vi "penning.vi"() -> ()   [LabVIEW 2014, in "Panels.lvlib"]
uses:
  Panels.lvlib
  CSlibraries-extern/DimLVEvent/DimIndicators/DimIndicators.lvlib
  CSlibraries/UtilityLib/UtilityLib.lvlib
  CSCore/CSSystem/CoreLib/CoreLib.lvlib
  CSlibraries/UtilityLib/UtilityLib.valueStatus.ctl
  Instance           1 15Saved   penning .vi
  CSCore/CSSystem/CoreLib/CoreLib.double 2 byte array.vi
  CSCore/CSSystem/CoreLib/CoreLib.string 2 byte array.vi
  CSlibraries-extern/DimLVEvent/LVDimInterface/LVDimInterface.lvlib
  CSCore/CSSystem/CoreLib/CoreLib.short 2 byte array.vi
  CSlibraries-extern/DimLVEvent/DimIndicators/DimIndicators.numericType.ctl
  CSCore/BaseProcess/BaseProcess.descriptor string definition.ctl
  CSCore/BaseProcess/BaseProcess.lvlib
  CSCore/CSSystem/CoreDefs/CoreDefs.rawDataType.ctl
  CSCore/CSSystem/CoreDefs/CoreDefs.call_type.ctl
  CSlibraries-extern/DimLVEvent/DimIndicators/DimIndicators.numericArrayType.ctl
  CSlibraries-extern/DimLVEvent/DimIndicators/DimIndicators.anyType.ctl
panel:
  in  "ListOfBases_Data":T1={"data"="NOLINK", "no link"=TRUE, "quality"=-1, "timeStamp"=0.0}
  in  "SetFileLocation_Data":T1={"data"="NOLINK", "no link"=TRUE, "quality"=-1, "timeStamp"=0.0}
  in  "call cluster in":T2={"Object"="", "Selector"="", "CallType"=enum."synchronous", "Async Object"="", "Async Selector"="", "Data Descriptor"="", "Data"=[], "Error #"=0, "Expire"=0}
  in  "CorrRingPara":dbl
  in  "CorrTubePara":dbl
  out "i ref out 2":refnum<vi>
  in  "i ref in":refnum<vi>
  in  "PT Viewer":bool
  in  "HypEndcapBEj":bool
  in  "HypRing":bool
  in  "HypCorrTubeBEj":bool
  in  "HypCorrTubeBInj":bool
  in  "HypCorrTubeAEj":bool
  in  "HypCorrTubeAInj":bool
  in  "HypEndcapAEj":bool
  in  "HypEndcapATrap":bool
  in  "HypEndcapAInj":bool
  in  "HypEndcapBInj":bool
  in  "HypEndcapBTrap":bool
  in  "HypEndcapAInj_SetValueInfoData":T5={"data"=[-121.4, 120.2, 1.0], "no link"=FALSE, "quality"=0, "timeStamp"=3268846606.097}
  in  "HypEndcapAInj_SetData":T5={"data"=[0.0, 0.0, 0.0, 0.0], "no link"=FALSE, "quality"=1, "timeStamp"=3268846604.644}
  in  "HypRing_MonData":T6={"data"=inf, "no link"=FALSE, "quality"=1, "timeStamp"=3268846606.097}
  in  "HypCorrRingB_MonData":T6={"data"=inf, "no link"=FALSE, "quality"=1, "timeStamp"=3268846606.097}
  in  "HypEndcapBTrap_MonData":T6={"data"=inf, "no link"=FALSE, "quality"=1, "timeStamp"=3268846606.082}
  in  "HypCorrTubeBTrap_MonData":T6={"data"=inf, "no link"=FALSE, "quality"=1, "timeStamp"=3268846606.082}
  in  "HypCorrRingA_MonData":T6={"data"=inf, "no link"=FALSE, "quality"=1, "timeStamp"=3268846606.097}
  in  "HypCorrTubeATrap_MonData":T6={"data"=inf, "no link"=FALSE, "quality"=1, "timeStamp"=3268846606.082}
  in  "HypEndcapATrap_MonData":T6={"data"=inf, "no link"=FALSE, "quality"=1, "timeStamp"=3268846606.097}
  in  "HypEndcapATrap_SetValueInfoData":T5={"data"=[-121.3, 120.5, 1.0], "no link"=FALSE, "quality"=0, "timeStamp"=3268846606.082}
  in  "HypEndcapAEj_SetValueInfoData":T5={"data"=[-120.0, 120.0, 1.0], "no link"=FALSE, "quality"=0, "timeStamp"=3268846606.097}
  in  "HypEndcapATrap_SetData":T5={"data"=[0.0, 0.0, 0.0, 0.0], "no link"=FALSE, "quality"=1, "timeStamp"=3268846604.629}
  in  "HypEndcapAEj_SetData":T5={"data"=[0.0, 0.0, 0.0, 0.0], "no link"=FALSE, "quality"=1, "timeStamp"=3268846604.644}
  in  "HypCorrTubeAEj_SetData":T5={"data"=[0.0, 0.0, 0.0, 0.0], "no link"=FALSE, "quality"=1, "timeStamp"=3268846604.644}
  in  "PenningBase_SetValueInfoData":T5={"data"=[0.0, 10.0, -1.0], "no link"=FALSE, "quality"=0, "timeStamp"=3268846606.097}
  in  "HypCorrTubeBInj_SetValueInfoData":T5={"data"=[-119.8, 119.3, 1.0], "no link"=FALSE, "quality"=0, "timeStamp"=3268846606.082}
  in  "PenningBase_SetData":T5={"data"=[0.0, 0.0, 0.0, 0.0], "no link"=FALSE, "quality"=1, "timeStamp"=3268846604.91}
  out "HypCorrTubeBTrap_Mon":dbl=inf caption="HypCorrTubeB_Mon" format="%.4f"
  out "HypCorrRingA_Mon":dbl=inf format="%.4f"
  out "HypRing_Mon":dbl=inf format="%.4f"
  in  "HypCorrTubeBEj_SetValueInfoData":T5={"data"=[-120.0, 120.0, 1.0], "no link"=FALSE, "quality"=0, "timeStamp"=3268846606.097}
  in  "HypCorrTubeBInj_SetData":T5={"data"=[0.0, 0.0, 0.0, 0.0], "no link"=FALSE, "quality"=1, "timeStamp"=3268846604.66}
  in  "HypEndcapBEj_SetValueInfoData":T5={"data"=[-120.0, 120.0, 1.0], "no link"=FALSE, "quality"=0, "timeStamp"=3268846606.082}
  in  "HypCorrTubeBEj_SetData":T5={"data"=[0.0, 0.0, 0.0, 0.0], "no link"=FALSE, "quality"=1, "timeStamp"=3268846604.676}
  out "HypCorrTubeATrap_Mon":dbl=inf format="%.4f"
  out "i ref out":refnum<vi>
  in  "Last Loaded File_Data":T1={"data"="NOLINK", "no link"=TRUE, "quality"=-1, "timeStamp"=0.0}
  out "FileUpToDate":bool=TRUE caption="Parameter Changed"
  in  "Close All Panels":bool
  in  "HypCorrTubeAInj_SetValueInfoData":T5={"data"=[-120.6, 119.6, 1.0], "no link"=FALSE, "quality"=0, "timeStamp"=3268846606.082}
  in  "HypRing_SetValueInfoData":T5={"data"=[-121.0, 119.7, 1.0], "no link"=FALSE, "quality"=0, "timeStamp"=3268846606.082}
  in  "CorrRingPara_SetValueInfoData":T5={"data"=[0.0, 1.0, -1.0], "no link"=FALSE, "quality"=0, "timeStamp"=3268846606.097}
  in  "CorrTubePara_SetValueInfoData":T5={"data"=[0.0, 1.0, -1.0], "no link"=FALSE, "quality"=0, "timeStamp"=3268846606.097}
  in  "HypEndcapBInj_SetValueInfoData":T5={"data"=[-120.5, 119.4, 1.0], "no link"=FALSE, "quality"=0, "timeStamp"=3268846606.097}
  in  "HypEndcapBTrap_SetValueInfoData":T5={"data"=[-120.6, 119.9, 1.0], "no link"=FALSE, "quality"=0, "timeStamp"=3268846606.082}
  in  "HypCorrTubeAEj_SetValueInfoData":T5={"data"=[-120.0, 120.0, 1.0], "no link"=FALSE, "quality"=0, "timeStamp"=3268846606.082}
  in  "HypEndcapBTrap_SetData":T5={"data"=[0.0, 0.0, 0.0, 0.0], "no link"=FALSE, "quality"=1, "timeStamp"=3268846604.644}
  in  "HypEndcapBInj_SetData":T5={"data"=[0.0, 0.0, 0.0, 0.0], "no link"=FALSE, "quality"=1, "timeStamp"=3268846604.66}
  in  "CorrTubePara_SetData":T5={"data"=[0.0, 0.0, 0.0, 0.0], "no link"=FALSE, "quality"=1, "timeStamp"=3268846604.894}
  in  "CorrRingPara_SetData":T5={"data"=[0.0, 0.0, 0.0, 0.0], "no link"=FALSE, "quality"=1, "timeStamp"=3268846604.894}
  in  "HypRing_SetData":T5={"data"=[0.0, 0.0, 0.0, 0.0], "no link"=FALSE, "quality"=1, "timeStamp"=3268846604.644}
  in  "HypCorrTubeAInj_SetData":T5={"data"=[0.0, 0.0, 0.0, 0.0], "no link"=FALSE, "quality"=1, "timeStamp"=3268846604.644}
  in  "HypEndcapBEj_SetData":T5={"data"=[0.0, 0.0, 0.0, 0.0], "no link"=FALSE, "quality"=1, "timeStamp"=3268846604.644}
  in  "call cluster in":T2={"Object"="", "Selector"="", "CallType"=enum."synchronous", "Async Object"="", "Async Selector"="", "Data Descriptor"="", "Data"=[], "Error #"=0, "Expire"=0}
  in  "PenningBase":dbl
  out "Last Loaded File":string
  in  "SetFileLocation":path=path "\\\\intranet\\Files/projects/lebit/Data Exchange/data/PenningControl"
  out "HypCorrRingB_Mon":dbl=inf format="%.4f"
  out "HypEndcapATrap_Mon":dbl=inf format="%.4f"
  out "HypEndcapBTrap_Mon":dbl=inf format="%.4f"
  # "Parameter changed, data file is no longer up-to-date."
  # "HypCorrRingA"
  # "HypCorrRingB"
  # "HypEndcapA"
  # "HypEndcapB"
  # "HypCorrTubeA"
  # "HypCorrTubeB"
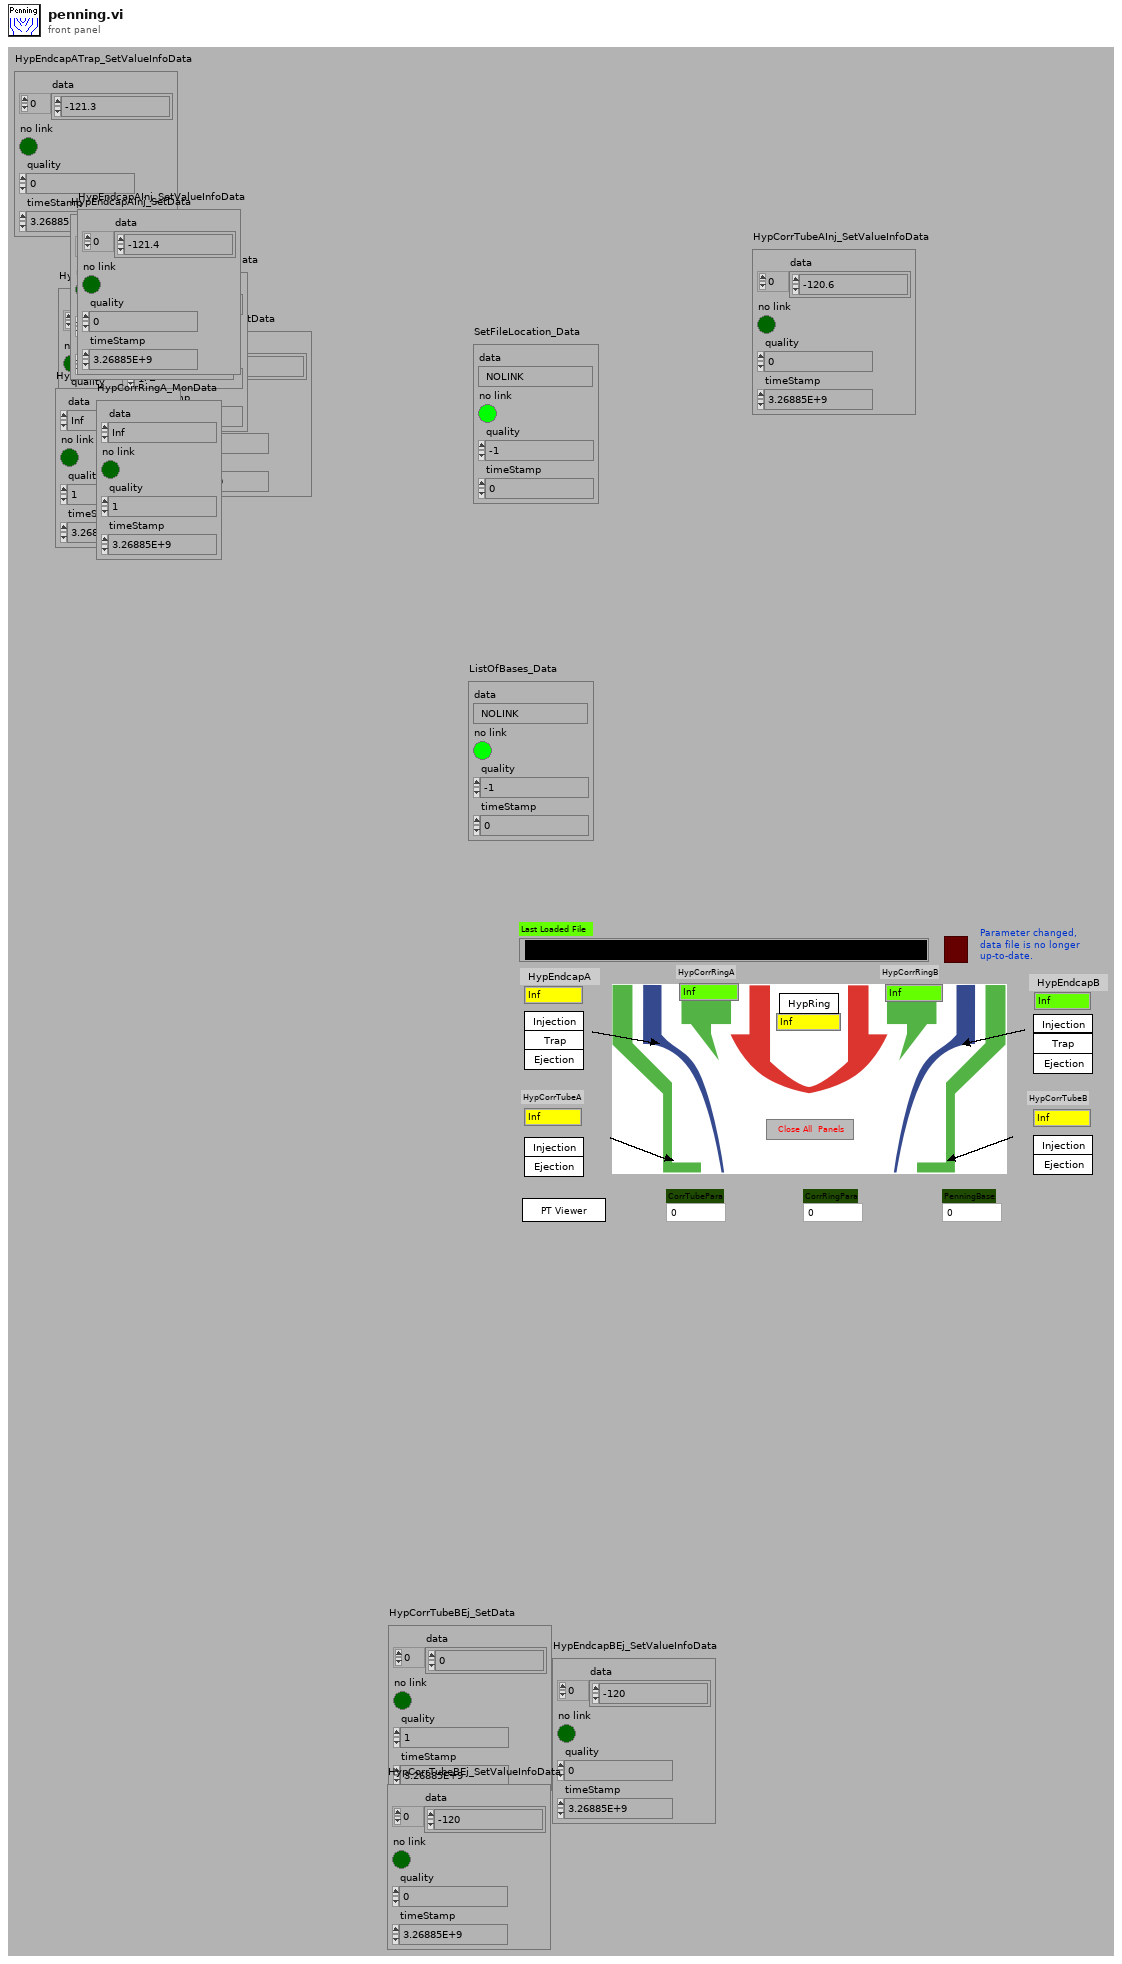
[diagram p1: front panel]
types:
  T1 = typedef "DimIndicators.lvlib/DimIndicators.anyType.ctl" = cluster{"data":string, "no link":bool, "quality":i32, "timeStamp":dbl}
  T2 = typedef "CoreDefs.call_type.ctl" = cluster{"Object":string, "Selector":string, "CallType":enum16{"simple", "synchronous", "asynchronous"}, "Async Object":string, "Async Selector":string, "Data Descriptor":T3, "Data":T4, "Error #":i32, "Expire":u32}
  T3 = typedef "BaseProcess.lvlib/BaseProcess.descriptor string definition.ctl" = string
  T4 = typedef "CoreDefs.rawDataType.ctl" = i8[]
  T5 = typedef "DimIndicators.lvlib/DimIndicators.numericArrayType.ctl" = cluster{"data":dbl[], "no link":bool, "quality":i32, "timeStamp":dbl}
  T6 = typedef "DimIndicators.lvlib/DimIndicators.numericType.ctl" = cluster{"data":dbl, "no link":bool, "quality":i32, "timeStamp":dbl}
  T7 = typedef "UtilityLib.lvlib/UtilityLib.valueStatus.ctl" = enum16{"no info available", "stand by/off", "on", "warning", "alarm/malfunction", "not implemented", "user action required", "important information", "system default", "control default", "indicator default", "button default"}
  T8 = cluster{"data":string, "no link":bool, "quality":i32, "timeStamp":dbl}
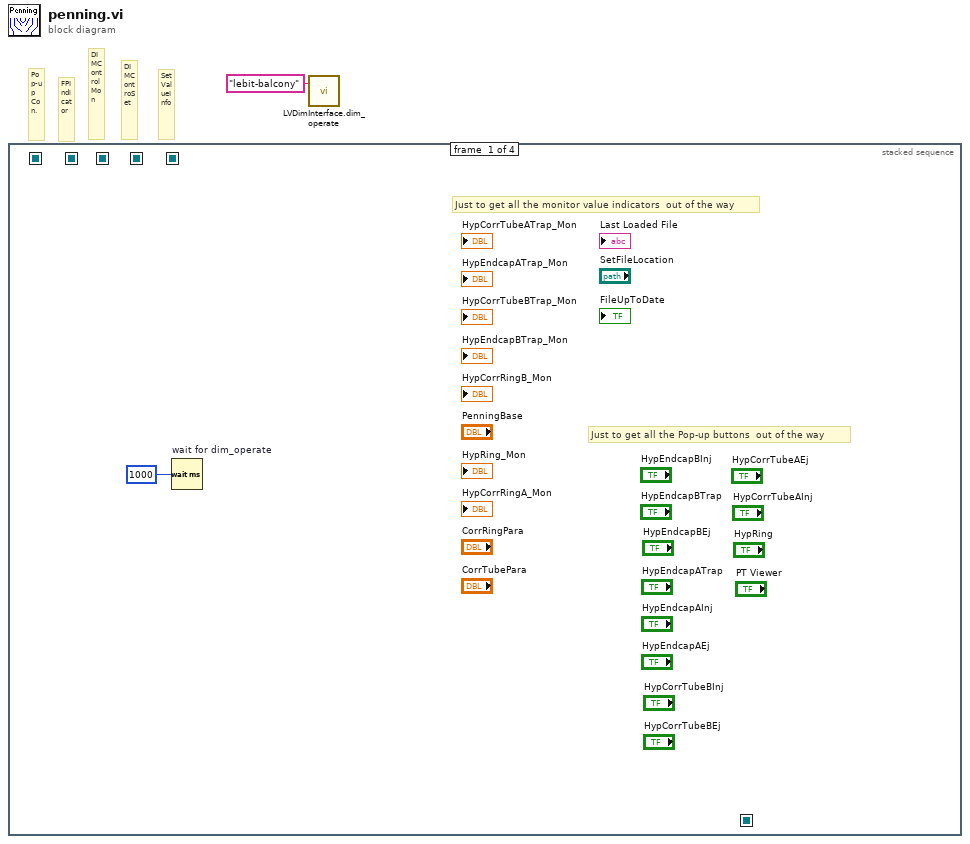
[diagram p0: block diagram]
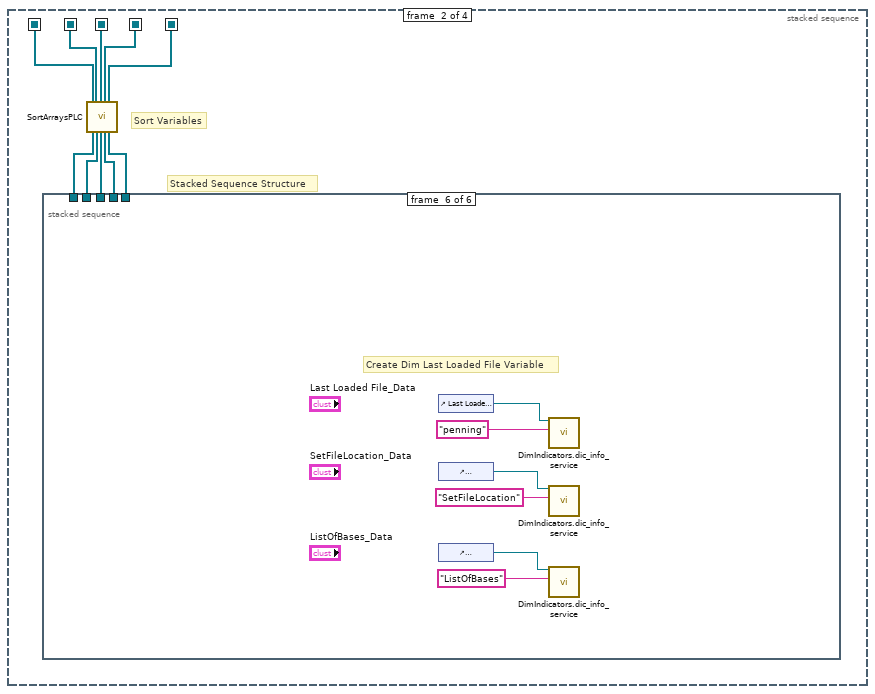
[diagram p2: hidden frame]
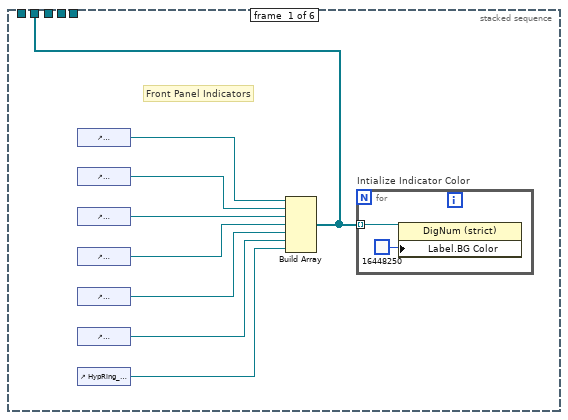
[diagram p3: hidden frame]
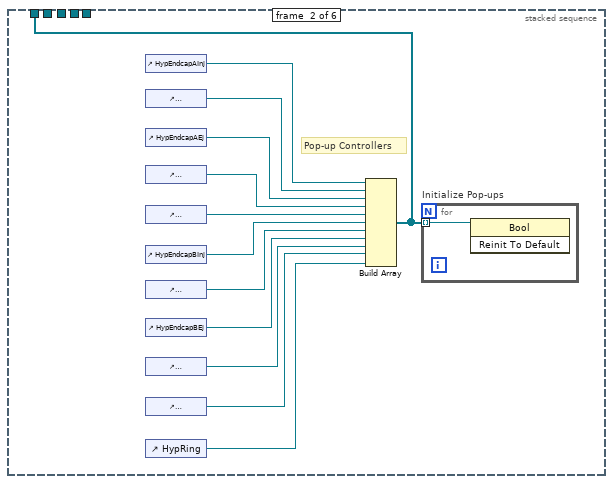
[diagram p4: hidden frame]
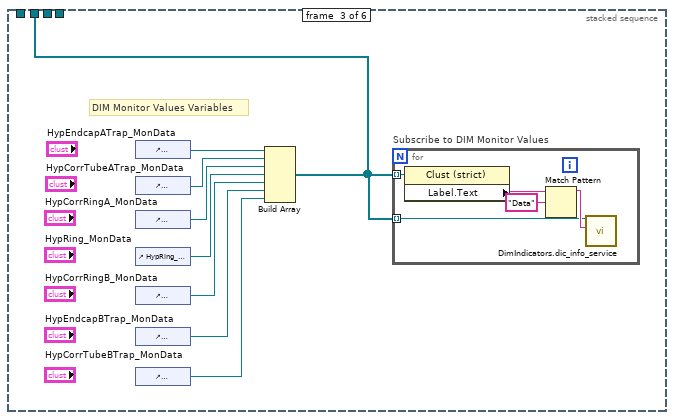
[diagram p5: hidden frame]
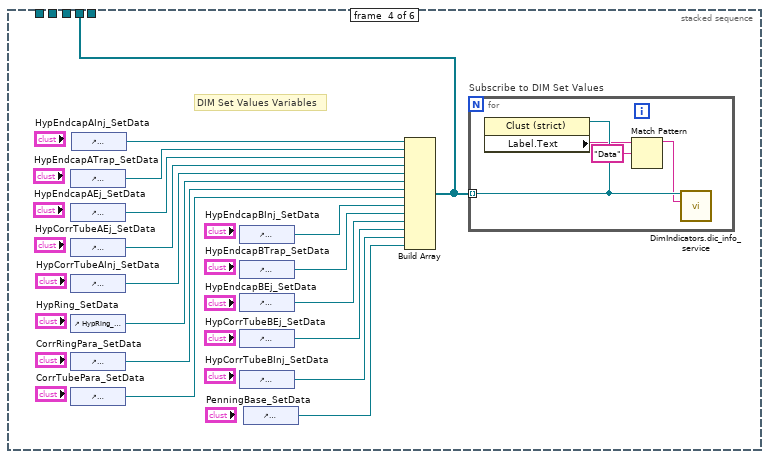
[diagram p6: hidden frame]
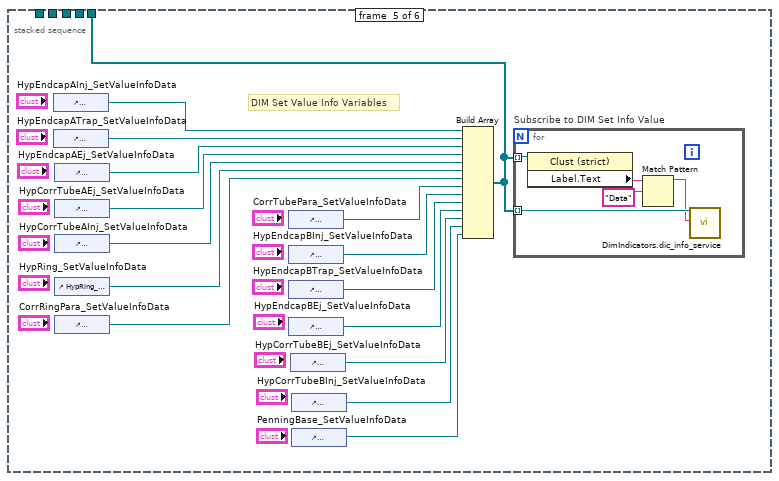
[diagram p7: hidden frame]
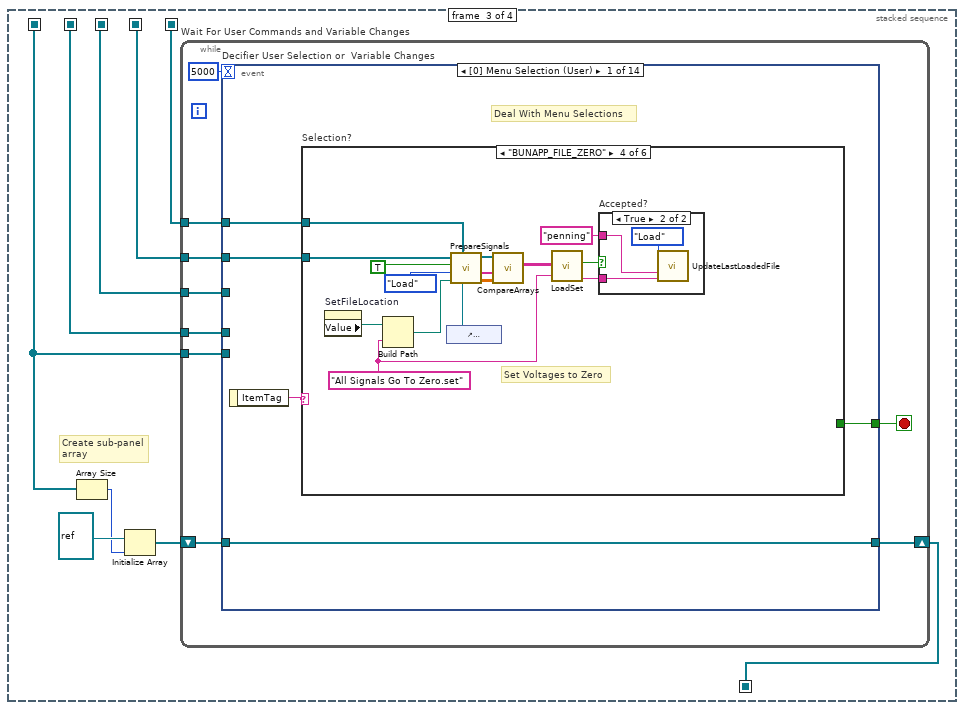
[diagram p8: hidden frame]
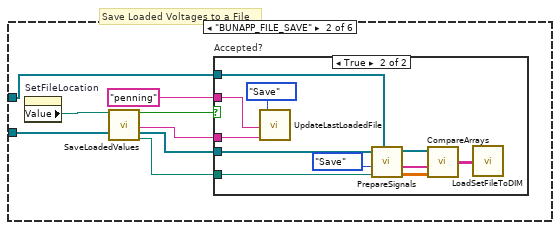
[diagram p10: hidden frame]
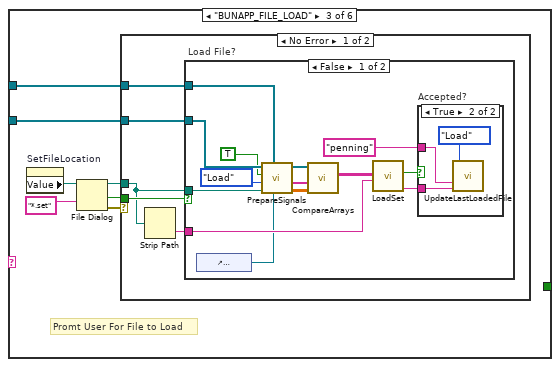
[diagram p12: hidden frame]
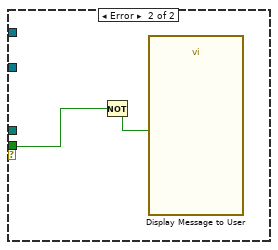
[diagram p15: hidden frame]
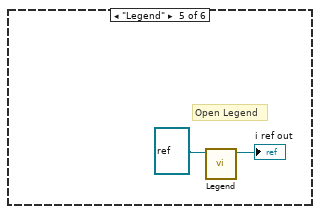
[diagram p17: hidden frame]
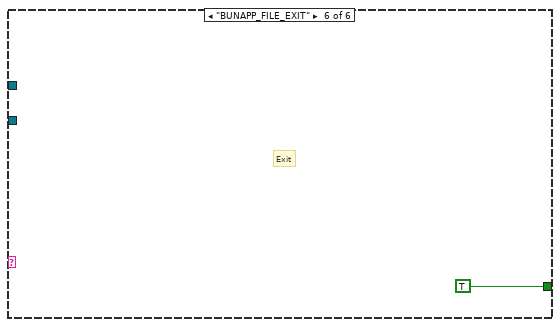
[diagram p18: hidden frame]
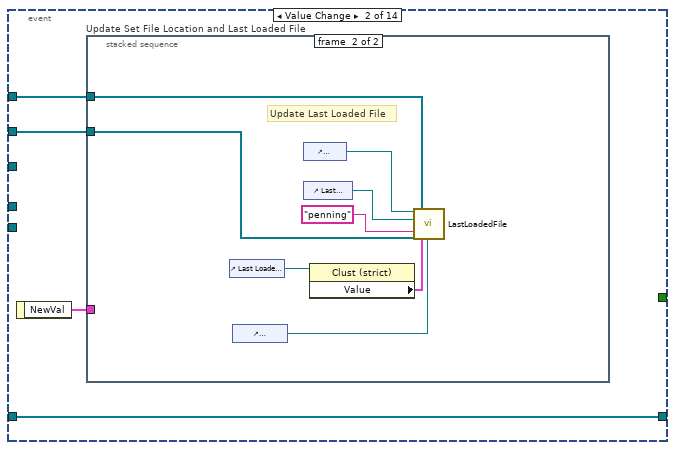
[diagram p19: hidden frame]
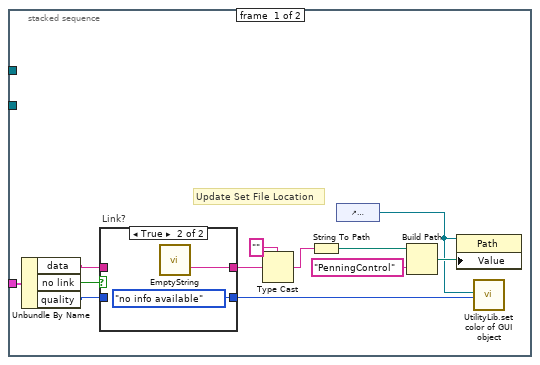
[diagram p20: hidden frame]
diagram:
  # "Pop-up Con."
  # "SetValueInfo"
  # "DIMControSet"
  # "DIMControlMon"
  # "FPIndicator"
  n1 = stacked-sequence {
    seq-local: [_ w10 _ _] -> [_ _ w99 _]
    seq-local: [_ w8 _ _] -> [_ _ w102 w396]
    seq-local: [_ _ w97 _] -> [_ _ _ w399]
    seq-local: [_ w9 _ _] -> [_ _ w96 w398]
    seq-local: [_ w12 _ _] -> [_ _ w95 w397]
    seq-local: [_ w11 _ _] -> [_ _ w94 _]
    frame #0 {
      # "Just to get all the Pop-up buttons  out of the way"
      # "Just to get all the monitor value indicators  out of the way"
      n2 = Wait (ms) "wait for dim_operate"(milliseconds to wait=u32 1000) -> ()  [unwired: 1 out]
    }
    frame #1 {
      # "Stacked Sequence Structure"
      # "Sort Variables"
      n3 = stacked-sequence {
        tunnel: [w13 _ _ _ _ _] -> w7
        tunnel: [_ w23 _ _ _ _] -> w6
        tunnel: [_ _ w36 _ _ _] -> w5
        tunnel: [_ _ _ w49 _ _] -> w4
        tunnel: [_ _ _ _ w68 _] -> w3
        frame #0 {
          # "Front Panel Indicators"
          n4 = control-ref of="HypEndcapATrap_Mon"() -> (w18:refnum<vi>)
          n5 = control-ref of="HypEndcapBTrap_Mon"() -> (w19:refnum<vi>)
          n6 = control-ref of="HypCorrTubeATrap_Mon"() -> (w17:refnum<vi>)
          n7 = control-ref of="HypCorrTubeBTrap_Mon"() -> (w16:refnum<vi>)
          n8 = control-ref of="HypCorrRingA_Mon"() -> (w20:refnum<vi>)
          n9 = control-ref of="HypCorrRingB_Mon"() -> (w15:refnum<vi>)
          n10 = control-ref of="HypRing_Mon"() -> (w14:refnum<vi>)
          n11 = Build Array(w18, w19, w17, w16, w20, w15, w14) -> (w13:refnum<vi>[])
          n12 = for "Intialize Indicator Color" {
            tunnel: w13 -> [w22] mode=indexing
            n13 = property class="DigNum (strict)"(reference=w22, "Label.BG Color"=u32 16448250 ("Color Box")) -> ()  [unwired: 1 in, 2 out]
          }
        }
        frame #1 {
          # "Pop-up Controllers"
          n14 = control-ref of="HypEndcapAInj"() -> (w34:refnum<vi>)
          n15 = control-ref of="HypEndcapATrap"() -> (w32:refnum<vi>)
          n16 = control-ref of="HypEndcapAEj"() -> (w31:refnum<vi>)
          n17 = control-ref of="HypCorrTubeAInj"() -> (w30:refnum<vi>)
          n18 = control-ref of="HypCorrTubeAEj"() -> (w29:refnum<vi>)
          n19 = control-ref of="HypEndcapBInj"() -> (w28:refnum<vi>)
          n20 = control-ref of="HypEndcapBTrap"() -> (w27:refnum<vi>)
          n21 = control-ref of="HypEndcapBEj"() -> (w26:refnum<vi>)
          n22 = control-ref of="HypCorrTubeBInj"() -> (w25:refnum<vi>)
          n23 = control-ref of="HypCorrTubeBEj"() -> (w24:refnum<vi>)
          n24 = control-ref of="HypRing"() -> (w33:refnum<vi>)
          n25 = Build Array(w34, w32, w31, w30, w29, w28, w27, w26, w25, w24, w33) -> (w23:refnum<vi>[])
          n26 = for "Initialize Pop-ups" {
            tunnel: w23 -> [w35] mode=indexing
            n27 = invoke class="Bool" method="Reinit To Default"(reference=w35) -> ()  [unwired: 2 in, 3 out]
          }
        }
        frame #2 {
          # "DIM Monitor Values Variables"
          n28 = control-ref of="HypEndcapATrap_MonData"() -> (w37:refnum<vi>)
          n29 = control-ref of="HypCorrTubeATrap_MonData"() -> (w39:refnum<vi>)
          n30 = control-ref of="HypCorrRingA_MonData"() -> (w38:refnum<vi>)
          n31 = control-ref of="HypRing_MonData"() -> (w43:refnum<vi>)
          n32 = control-ref of="HypCorrRingB_MonData"() -> (w42:refnum<vi>)
          n33 = control-ref of="HypEndcapBTrap_MonData"() -> (w41:refnum<vi>)
          n34 = control-ref of="HypCorrTubeBTrap_MonData"() -> (w40:refnum<vi>)
          n35 = Build Array(w37, w39, w38, w43, w42, w41, w40) -> (w36:refnum<vi>[])
          n36 = for "Subscribe to DIM Monitor Values" {
            tunnel: w36 -> [w45] mode=indexing
            tunnel: w36 -> [w44] mode=indexing
            n37 = property class="Clust (strict)"(reference=w45) -> ("Label.Text"=w47:string)  [unwired: 1 in, 2 out]
            n38 = Match Pattern(string=w47, regular expression="Data") -> (before substring=w46:string)  [unwired: 1 in, 3 out]
            n39 = call "DimIndicators.dic_info_service.vi"("controlRef"=w44, "serviceName"=w46) -> ()  [unwired: 16 in, 2 out]
          }
        }
        frame #3 {
          # "DIM Set Values Variables"
          n40 = control-ref of="HypEndcapATrap_SetData"() -> (w53:refnum<vi>)
          n41 = control-ref of="HypEndcapAEj_SetData"() -> (w54:refnum<vi>)
          n42 = control-ref of="HypCorrTubeAEj_SetData"() -> (w55:refnum<vi>)
          n43 = control-ref of="HypCorrTubeAInj_SetData"() -> (w63:refnum<vi>)
          n44 = control-ref of="HypRing_SetData"() -> (w62:refnum<vi>)
          n45 = control-ref of="CorrRingPara_SetData"() -> (w61:refnum<vi>)
          n46 = control-ref of="CorrTubePara_SetData"() -> (w50:refnum<vi>)
          n47 = control-ref of="HypEndcapAInj_SetData"() -> (w51:refnum<vi>)
          n48 = control-ref of="HypEndcapBInj_SetData"() -> (w60:refnum<vi>)
          n49 = control-ref of="HypEndcapBTrap_SetData"() -> (w59:refnum<vi>)
          n50 = control-ref of="HypEndcapBEj_SetData"() -> (w58:refnum<vi>)
          n51 = control-ref of="HypCorrTubeBEj_SetData"() -> (w57:refnum<vi>)
          n52 = control-ref of="HypCorrTubeBInj_SetData"() -> (w56:refnum<vi>)
          n53 = control-ref of="PenningBase_SetData"() -> (w52:refnum<vi>)
          n54 = Build Array(w51, w53, w54, w55, w63, w62, w61, w50, w60, w59, w58, w57, w56, w52) -> (w49:refnum<vi>[])
          n55 = for "Subscribe to DIM Set Values" {
            tunnel: w49 -> [w67] mode=indexing
            n56 = property class="Clust (strict)"(reference=w67) -> ("Label.Text"=w66:string)  [unwired: 1 in, 2 out]
            n57 = Match Pattern(string=w66, regular expression="Data") -> (before substring=w64:string)  [unwired: 1 in, 3 out]
            n58 = call "DimIndicators.dic_info_service.vi"("controlRef"=w67, "serviceName"=w64) -> ()  [unwired: 16 in, 2 out]
          }
        }
        frame #4 {
          # "DIM Set Value Info Variables"
          n59 = control-ref of="HypEndcapAInj_SetValueInfoData"() -> (w69:refnum<vi>)
          n60 = control-ref of="HypEndcapATrap_SetValueInfoData"() -> (w73:refnum<vi>)
          n61 = control-ref of="HypEndcapAEj_SetValueInfoData"() -> (w72:refnum<vi>)
          n62 = control-ref of="HypCorrTubeAEj_SetValueInfoData"() -> (w82:refnum<vi>)
          n63 = control-ref of="HypCorrTubeAInj_SetValueInfoData"() -> (w81:refnum<vi>)
          n64 = control-ref of="HypRing_SetValueInfoData"() -> (w80:refnum<vi>)
          n65 = control-ref of="CorrRingPara_SetValueInfoData"() -> (w79:refnum<vi>)
          n66 = control-ref of="CorrTubePara_SetValueInfoData"() -> (w78:refnum<vi>)
          n67 = control-ref of="HypEndcapBInj_SetValueInfoData"() -> (w77:refnum<vi>)
          n68 = control-ref of="HypEndcapBTrap_SetValueInfoData"() -> (w76:refnum<vi>)
          n69 = control-ref of="HypEndcapBEj_SetValueInfoData"() -> (w75:refnum<vi>)
          n70 = control-ref of="HypCorrTubeBEj_SetValueInfoData"() -> (w74:refnum<vi>)
          n71 = control-ref of="HypCorrTubeBInj_SetValueInfoData"() -> (w71:refnum<vi>)
          n72 = control-ref of="PenningBase_SetValueInfoData"() -> (w70:refnum<vi>)
          n73 = Build Array(w69, w73, w72, w82, w81, w80, w79, w78, w77, w76, w75, w74, w71, w70) -> (w68:refnum<vi>[])
          n74 = for "Subscribe to DIM Set Info Value" {
            tunnel: w68 -> [w83] mode=indexing
            tunnel: w68 -> [w87] mode=indexing
            n75 = property class="Clust (strict)"(reference=w83) -> ("Label.Text"=w86:string)  [unwired: 1 in, 2 out]
            n76 = Match Pattern(string=w86, regular expression="Data") -> (before substring=w84:string)  [unwired: 1 in, 3 out]
            n77 = call "DimIndicators.dic_info_service.vi"("controlRef"=w87, "serviceName"=w84) -> ()  [unwired: 16 in, 2 out]
          }
        }
        frame #5 {
          # "Create Dim Last Loaded File Variable"
          n78 = control-ref of="Last Loaded File_Data"() -> (w91:refnum<vi>)
          n79 = control-ref of="SetFileLocation_Data"() -> (w93:refnum<vi>)
          n80 = control-ref of="ListOfBases_Data"() -> (w89:refnum<vi>)
          n81 = call "DimIndicators.dic_info_service.vi"("controlRef"=w91, "serviceName"="penning" ("string")) -> ()  [unwired: 16 in, 2 out]
          n82 = call "DimIndicators.dic_info_service.vi"("controlRef"=w93, "serviceName"="SetFileLocation" ("string")) -> ()  [unwired: 16 in, 2 out]
          n83 = call "DimIndicators.dic_info_service.vi"("controlRef"=w89, "serviceName"="ListOfBases" ("string")) -> ()  [unwired: 16 in, 2 out]
        }
      }
      n84 = call "SortArraysPLC.vi"("Pop-up Con."=w6, "FPIndicator in"=w7, "DIMControlMon"=w5, "DIMControSet"=w4, "SetValueInfo"=w3) -> ("Pop-up Con. out"=w11:refnum<vi>[], "FPIndicator out"=w10:refnum<vi>[], "DIMControlMon out"=w8:refnum<vi>[], "DIMControSet out"=w9:refnum<vi>[], "SetValueInfo out"=w12:refnum<vi>[])  [unwired: 18 in]
    }
    frame #2 {
      # "Create sub-panel\narray"
      n85 = Array Size(array=w94) -> (size(s)=w98:i32)
      n86 = Initialize Array(refnum<vi> refnum ("vi reference"), w98) -> (w101:refnum<vi>[])
      n87 = while "Wait For User Commands and Variable Changes" {
        tunnel: w102 -> [w110]
        tunnel: w99 -> [w109]
        shift-right: [w107] -> w97
        shift-left: w101 -> [w108]
        tunnel: w96 -> [w106]
        tunnel: w95 -> [w105]
        tunnel: w94 -> [w103]
        stop <- w111 stop-if-true
        n88 = event "Decifier User Selection or  Variable Changes" shown="[0] Menu Selection (User)" {
          selector: _ -> [_ _ _ _ _ _ _ _ _ _ _ _ _ _]
          dyn-events: _ -> [_ _ _ _ _ _ _ _ _ _ _ _ _ _]
          timeout: 5000 -> [_ _ _ _ _ _ _ _ _ _ _ _ _ _]
          tunnel: [w113 _ _ _ _ _ _ _ _ _ _ _ _ TRUE ("stop")] -> w111
          tunnel: w110 -> [_ _ _ _ _ _ w276 _ _ _ _ _ _ w370]
          tunnel: w109 -> [_ _ _ _ _ _ w275 _ _ _ _ _ _ _]
          tunnel: w108 -> [w116 w189 w224 w225 w235 w258 w278 w307 w312 w324 w354 w361 w367 w369]
          tunnel: [w116 w189 w224 w225 w235 w258 w278 w307 w312 w324 w352 w359 w367 _] -> w107
          tunnel: w106 -> [w114 w190 w221 _ w236 w256 _ _ w310 w315 _ _ _ w371]
          tunnel: w105 -> [w112 w188 w218 _ w237 _ _ _ _ _ _ _ _ w372]
          tunnel: w103 -> [_ _ _ _ _ _ _ _ _ _ w349 _ _ _]
          event Menu Selection (User) {
            # "Deal With Menu Selections"
            n89 = event-data() -> ("ItemTag"=w115:string)  [unwired: 1 in]
            n90 = case "Selection?" shown="\"BUNAPP_FILE_ZERO\"" w115 {
              tunnel: w114 -> [_ w121 w141 w181 _ _]
              tunnel: [_ _ _ _ _ TRUE ("stop")] -> w113
              tunnel: w112 -> [_ w117 w136 w168 _ _]
              frame "False", Default {
              }
              frame "BUNAPP_FILE_SAVE" {
                # "Save Loaded Voltages to a File"
                n91 = property on="SetFileLocation" class="Path"() -> ("Value"=w122:path)  [unwired: 2 in, 2 out]
                n92 = call "SaveLoadedValues.vi"("Panel Location?"=w122, "DIMControlSet in"=w121) -> ("File Saved?"=w123:bool, "File Name"=w120:string, "DIMControlSet out"=w118:refnum<vi>[], "Path"=w119:path)  [unwired: 14 in]
                n93 = case "Accepted?" shown="True" w123 {
                  tunnel: w120 -> [_ w133]
                  tunnel: "penning" ("string") -> [_ w135]
                  tunnel: w118 -> [_ w134]
                  tunnel: w119 -> [_ w132]
                  tunnel: w117 -> [_ w126]
                  frame False {
                  }
                  frame True {
                    n94 = call "UpdateLastLoadedFile.vi"("LoadOrSave"=enum16{"Load", "Save"}."Save", "GUIName"=w135, "FileNameIn"=w133) -> ()  [unwired: 13 in]
                    n95 = call "PrepareSignals.vi"("SetValueInfo in"=w126, "setfile path"=w132, "Enum"=enum16{"Save", "Load"}."Save", "DIMControSet in"=w134) -> ("indexed loaded Array"=w130:dbl[][], "Name Array"=w131:string[], "DIMControSet out"=w129:refnum<vi>[])  [unwired: 5 in]
                    n96 = call "CompareArrays.vi"("indexed loaded Array"=w130, "Name Array"=w131, "DIMControSet"=w129) -> ("Table for loading values"=w128:string[][])  [unwired: 4 in]
                    n97 = call "LoadSetFileToDIM.vi"("output array"=w128) -> ()  [unwired: 2 in]
                  }
                }
              }
              frame "BUNAPP_FILE_LOAD" {
                # "Promt User For File to Load"
                n98 = property on="SetFileLocation" class="Path"() -> ("Value"=w138:path)  [unwired: 2 in, 2 out]
                n99 = File Dialog(6:"*.set" ("pattern (all files)"), 11:w138) -> (0:w137:errorcluster, 1:w142:bool, 3:w139:path)  [unwired: 5 in, 1 out]
                n100 = case shown="No Error" w137 {
                  tunnel: w142 -> [w147 w165]
                  tunnel: w141 -> [w146 _]
                  tunnel: w139 -> [w144 _]
                  tunnel: w136 -> [w143 _]
                  frame No Error {
                    n101 = Strip Path(path=w144) -> (name=w145:string)  [unwired: 1 out]
                    n102 = case "Load File?" shown="False" w147 {
                      tunnel: w146 -> [w161 _]
                      tunnel: w145 -> [w155 _]
                      tunnel: w144 -> [w156 _]
                      tunnel: w143 -> [w149 _]
                      frame False {
                        n103 = control-ref of="ListOfBases_Data"() -> (w148:refnum<vi>)
                        n104 = call "PrepareSignals.vi"("ListOfBases_Data"=w148, "SetValueInfo in"=w149, "setfile path"=w156, "Enum"=enum16{"Save", "Load"}."Load", "Display Message to \nUser"=TRUE ("Display Message to \nUser"), "DIMControSet in"=w161) -> ("indexed loaded Array"=w159:dbl[][], "Name Array"=w158:string[], "DIMControSet out"=w160:refnum<vi>[])  [unwired: 3 in]
                        n105 = call "CompareArrays.vi"("indexed loaded Array"=w159, "Name Array"=w158, "DIMControSet"=w160) -> ("Table for loading values"=w157:string[][])  [unwired: 4 in]
                        n106 = call "LoadSet.vi"("File Name In"=w155, "output array"=w157) -> ("File Name out"=w154:string, "Accepted"=w153:bool)  [unwired: 8 in]
                        n107 = case "Accepted?" shown="True" w153 {
                          tunnel: w154 -> [_ w164]
                          tunnel: "penning" ("string") -> [_ w163]
                          frame False {
                          }
                          frame True {
                            n108 = call "UpdateLastLoadedFile.vi"("LoadOrSave"=enum16{"Load", "Save"}."Load", "GUIName"=w163, "FileNameIn"=w164) -> ()  [unwired: 13 in]
                          }
                        }
                      }
                      frame True {
                      }
                    }
                  }
                  frame Error {
                    n109 = Not(x=w165) -> (.not. x?=w166:bool)
                    n110 = call "Display Message to User"("Enable"=w166) -> ()  [unwired: 9 in, 2 out]
                  }
                }
              }
              frame "BUNAPP_FILE_ZERO" {
                w172 = "All Signals Go To Zero.set" ("File Name")
                # "Set Voltages to Zero"
                n111 = property on="SetFileLocation" class="Path"() -> ("Value"=w170:path)  [unwired: 2 in, 2 out]
                n112 = Build Path(base path=w170, name or relative path=w172) -> (appended path=w171:path)
                n113 = control-ref of="ListOfBases_Data"() -> (w167:refnum<vi>)
                n114 = call "PrepareSignals.vi"("ListOfBases_Data"=w167, "SetValueInfo in"=w168, "setfile path"=w171, "Enum"=enum16{"Save", "Load"}."Load", "Display Message to \nUser"=TRUE ("Display Message to \nUser"), "DIMControSet in"=w181) -> ("indexed loaded Array"=w179:dbl[][], "Name Array"=w178:string[], "DIMControSet out"=w180:refnum<vi>[])  [unwired: 3 in]
                n115 = call "CompareArrays.vi"("indexed loaded Array"=w179, "Name Array"=w178, "DIMControSet"=w180) -> ("Table for loading values"=w177:string[][])  [unwired: 4 in]
                n116 = call "LoadSet.vi"("File Name In"=w172, "output array"=w177) -> ("File Name out"=w175:string, "Accepted"=w176:bool)  [unwired: 8 in]
                n117 = case "Accepted?" shown="True" w176 {
                  tunnel: w175 -> [_ w184]
                  tunnel: "penning" ("string") -> [_ w183]
                  frame False {
                  }
                  frame True {
                    n118 = call "UpdateLastLoadedFile.vi"("LoadOrSave"=enum16{"Load", "Save"}."Load", "GUIName"=w183, "FileNameIn"=w184) -> ()  [unwired: 13 in]
                  }
                }
              }
              frame "Legend" {
                # "Open Legend"
                n119 = call "Legend.vi"("i ref in"=refnum<vi> refnum) -> ("i ref out"=→"i ref out":refnum<vi>)  [unwired: 10 in]
              }
              frame "BUNAPP_FILE_EXIT" {
                # "Exit"
              }
            }
          }
          event Value Change {
            n120 = event-data() -> ("NewVal"=w191:T1)  [unwired: 1 in]
            n121 = stacked-sequence "Update Set File Location and Last Loaded File" {
              tunnel: w191 -> [w193 _]
              tunnel: w190 -> [_ w214]
              tunnel: w188 -> [_ w210]
              frame #0 {
                # "Update Set File Location"
                n122 = Unbundle By Name(w193) -> ("data"=w202:string, "no link"=w201:bool, "quality"=w200:i32)
                n123 = case "Link?" shown="True" w201 {
                  tunnel: w200 -> [w206 _]
                  tunnel: [w205 UtilityLib.valueStatus."no info available" ("valueStatus")] -> w203
                  tunnel: w202 -> [w204 _]
                  tunnel: [w204 w207] -> w198
                  frame False {
                    n124 = call "CoreLib.quality 2 status.vi"("quality"=w206) -> ("valueStatus"=w205:T7)  [unwired: 18 in]
                  }
                  frame True {
                    n125 = call "EmptyString.vi"() -> ("String"=w207:string)
                  }
                }
                n126 = Type Cast(type="" ("regular expression"), x=w198) -> (*(type *) &x=w197:string)
                n127 = String To Path(string=w197) -> (path=w194:path)
                n128 = control-ref of="SetFileLocation"() -> (w192:refnum<vi>)
                n129 = Build Path(base path=w194, name or relative path="PenningControl") -> (appended path=w195:path)
                n130 = property class="Path"(reference=w192, "Value"=w195) -> ()  [unwired: 1 in, 2 out]
                n131 = call "UtilityLib.set color of GUI object.vi"("GUI object Ref"=w192, "valueStatus"=w203) -> ()  [unwired: 17 in, 1 out]
              }
              frame #1 {
                # "Update Last Loaded File"
                n132 = control-ref of="Last Loaded File_Data"() -> (w215:refnum<vi>)
                n133 = control-ref of="ListOfBases_Data"() -> (w209:refnum<vi>)
                n134 = control-ref of="SetFileLocation"() -> (w212:refnum<vi>)
                n135 = control-ref of="Last Loaded File"() -> (w213:refnum<vi>)
                n136 = property class="Clust (strict)"(reference=w215) -> ("Value"=w216:T8)  [unwired: 1 in, 2 out]
                n137 = call "LastLoadedFile.vi"("SetFileLocation"=w212, "Last Loaded File"=w213, "GUIName"="penning" ("string"), "DIMControSet in"=w214, "SetValueInfo in"=w210, "NewVal"=w216, "ListOfBases_Data"=w209) -> ()  [unwired: 13 in]
              }
            }
          }
          event Value Change {
            # "Update Last Loaded File"
            n138 = event-data() -> ("NewVal"=w223:T1)  [unwired: 1 in]
            n139 = control-ref of="SetFileLocation"() -> (w220:refnum<vi>)
            n140 = control-ref of="Last Loaded File"() -> (w219:refnum<vi>)
            n141 = control-ref of="ListOfBases_Data"() -> (w217:refnum<vi>)
            n142 = call "LastLoadedFile.vi"("SetFileLocation"=w220, "Last Loaded File"=w219, "GUIName"="penning" ("string"), "DIMControSet in"=w221, "SetValueInfo in"=w218, "NewVal"=w223, "ListOfBases_Data"=w217) -> ()  [unwired: 13 in]
          }
          event "PT Viewer": Value Change {
            # "Open PT Viewer"
            n143 = event-data() -> ("CtlRef"=w226:refnum<vi>)  [unwired: 1 in, 5 out]
            n144 = invoke on="Initialize to Default" class="Bool" method="Reinit To Default"(reference=w226) -> ()  [unwired: 2 in, 3 out]
            n145 = call "ptspecial.vi"("i ref in"="i ref in") -> ("i ref out"=→"i ref out 2":refnum<vi>)  [unwired: 10 in]
          }
          event "PenningBase": Value Change {
            w229 = "PenningBase" ("string")
            # "Is Base in Range?"
            # "Update  Set Values"
            n146 = event-data() -> ("NewVal"=w232:dbl, "OldVal"=w231:dbl)  [unwired: 1 in, 4 out]
            n147 = control-ref of="ListOfBases_Data"() -> (w230:refnum<vi>)
            n148 = call "IsBaseInRange.vi"("SetValueInfo"=w237, "DIMControSet"=w236, "ListOfBases_Data"=w230, "NewVal in"=w232, "Base Name"=w229) -> ("NewVal Out"=w233:dbl, "In Range"=w234:bool)  [unwired: 13 in]
            n149 = case "Base In Range?" shown="True" w234 {
              tunnel: w233 -> [_ w242]
              tunnel: w231 -> [w238 _]
              tunnel: w229 -> [_ w239]
              frame False {
                n150 = property on="PenningBase" class="DigNum (strict)"("Value"=w238) -> ()  [unwired: 2 in, 2 out]
              }
              frame True {
                n151 = call-poly "CoreLib.data 2 byte array.vi"("i16"=i16 1 ("element")) -> ("byteArray out"=w241:T4)  [unwired: 18 in]
                n152 = property on="PenningBase" class="DigNum (strict)"("Value"=w242) -> ()  [unwired: 2 in, 2 out]
                n153 = call-poly "CoreLib.data 2 byte array.vi"("byteArray"=w241, "f64"=w242) -> ("byteArray out"=w246:T4)  [unwired: 17 in]
                n154 = Flatten To String(anything=TRUE) -> (data string=w245:string)  [unwired: 3 in, 2 out]
                n155 = Concatenate Strings("SetPLC" ("string"), w239) -> (w251:string)
                n156 = call-poly "CoreLib.data 2 byte array.vi"("byteArray"=w246, "string"=w245) -> ("byteArray out"=w243:T4)  [unwired: 17 in]
                n157 = Bundle By Name(cluster="call cluster in", "Object"="PLC", "Selector"=w251, "CallType"=enum16{"simple", "synchronous", "asynchronous"}."simple", "Data"=w243) -> (w248:T2)
                n158 = call "CoreLib.call process.vi"("call cluster in"=w248) -> ()  [unwired: 13 in, 2 out]
              }
            }
          }
          event Value Change {
            # "Update bunBase Set Value"
            n159 = event-data() -> ("CtlRef"=w255:refnum<vi>, "NewVal"=w260:T5)  [unwired: 1 in, 4 out]
            n160 = Unbundle By Name(w260) -> ("data"=w261:dbl[], "no link"=w262:bool, "quality"=w264:i32)
            n161 = case "Link?" shown="False" w262 {
              tunnel: w264 -> [w266 _]
              tunnel: [w265 UtilityLib.valueStatus."no info available" ("valueStatus")] -> w263
              tunnel: w261 -> [w268 _]
              tunnel: [w267 inf] -> w257
              frame False {
                n162 = call "CoreLib.quality 2 status.vi"("quality"=w266) -> ("valueStatus"=w265:T7)  [unwired: 18 in]
                n163 = Index Array(array=w268, index=0) -> (element=w267:dbl)
              }
              frame True {
              }
            }
            n164 = property on="FileUpToDate" class="Bool (strict)"() -> ("Value"=w253:bool)  [unwired: 2 in, 2 out]
            n165 = call "FileUpToDate.vi"("FileUpToDate in"=w253, "DIMControSet out"=w256, "CtlRef"=w255) -> ("FileUpToDate out"=w254:bool)  [unwired: 16 in]
            n166 = property on="FileUpToDate" class="Bool (strict)"("Value"=w254) -> ()  [unwired: 2 in, 2 out]
            n167 = control-ref of="PenningBase"() -> (w259:refnum<vi>)
            n168 = property on="PenningBase" class="DigNum (strict)"("Value"=w257) -> ()  [unwired: 2 in, 2 out]
            n169 = call "UtilityLib.set color of GUI object.vi"("GUI object Ref"=w259, "valueStatus"=w263) -> ()  [unwired: 17 in, 1 out]
          }
          event Value Change {
            # "Find Monitor Value Index"
            # "Updating a Monitor Value"
            n170 = event-data() -> ("CtlRef"=w274:refnum<vi>, "NewVal"=w279:T6)  [unwired: 1 in, 4 out]
            n171 = Search 1D Array(1D array=w276, element=w274) -> (index of element=w277:i32)  [unwired: 1 in]
            n172 = Index Array(array=w275, index=w277) -> (element=w272:refnum<vi>)
            n173 = Not A Number/Path/Refnum?(number/path/refnum=w272) -> (NaN/Path/Refnum?=w273:bool)
            n174 = case "Indicator exists?" shown="False" w273 {
              tunnel: w279 -> [_ w286]
              tunnel: w272 -> [_ w280]
              frame True {
              }
              frame False {
                n175 = Unbundle By Name(w286) -> ("data"=w282:dbl, "no link"=w283:bool, "quality"=w285:i32)
                n176 = case shown="False" w283 {
                  tunnel: w285 -> [w289 _]
                  tunnel: [w288 UtilityLib.valueStatus."no info available" ("valueStatus")] -> w284
                  tunnel: w282 -> [w287 _]
                  tunnel: [w287 inf] -> w281
                  frame False {
                    n177 = call "CoreLib.quality 2 status.vi"("quality"=w289) -> ("valueStatus"=w288:T7)  [unwired: 18 in]
                  }
                  frame True {
                  }
                }
                n178 = property class="DigNum (strict)"(reference=w280, "Value"=w281) -> ()  [unwired: 1 in, 2 out]
                n179 = call "TextColor.vi"("valueStatus"=w284, "reference"=w280) -> ()  [unwired: 10 in]
              }
            }
          }
          event "CorrTubePara", "CorrRingPara": Value Change {
            # "Update CorrTubePara or CorrRingPara"
            n180 = event-data() -> ("CtlRef"=w294:refnum<vi>, "NewVal"=w292:dbl)  [unwired: 1 in, 4 out]
            n181 = property class="DigNum (strict)"(reference=w294) -> ("Label.Text"=w293:string)  [unwired: 1 in, 2 out]
            n182 = call-poly "CoreLib.data 2 byte array.vi"("i16"=i16 1 ("element")) -> ("byteArray out"=w296:T4)  [unwired: 18 in]
            n183 = call-poly "CoreLib.data 2 byte array.vi"("byteArray"=w296, "f64"=w292) -> ("byteArray out"=w300:T4)  [unwired: 17 in]
            n184 = Flatten To String(anything=TRUE) -> (data string=w299:string)  [unwired: 3 in, 2 out]
            n185 = Concatenate Strings("SetPLC" ("string"), w293) -> (w305:string)
            n186 = call-poly "CoreLib.data 2 byte array.vi"("byteArray"=w300, "string"=w299) -> ("byteArray out"=w297:T4)  [unwired: 17 in]
            n187 = Bundle By Name(cluster="call cluster in", "Object"="PLC", "Selector"=w305, "CallType"=enum16{"simple", "synchronous", "asynchronous"}."simple", "Data"=w297) -> (w302:T2)
            n188 = call "CoreLib.call process.vi"("call cluster in"=w302) -> ()  [unwired: 13 in, 2 out]
          }
          event Value Change {
            n189 = event-data() -> ("CtlRef"=w311:refnum<vi>)  [unwired: 1 in, 5 out]
            n190 = property on="FileUpToDate" class="Bool (strict)"() -> ("Value"=w309:bool)  [unwired: 2 in, 2 out]
            n191 = call "FileUpToDate.vi"("FileUpToDate in"=w309, "DIMControSet out"=w310, "CtlRef"=w311) -> ("FileUpToDate out"=w308:bool)  [unwired: 16 in]
            n192 = property on="FileUpToDate" class="Bool (strict)"("Value"=w308) -> ()  [unwired: 2 in, 2 out]
          }
          event Value Change {
            n193 = event-data() -> ("CtlRef"=w314:refnum<vi>, "NewVal"=w323:T5)  [unwired: 1 in, 2 out]
            n194 = Unbundle By Name(w323) -> ("data"=w322:dbl[], "no link"=w318:bool, "quality"=w317:i32)
            n195 = property class="Clust (strict)"(reference=w314) -> ("Label.Text"=w320:string)  [unwired: 1 in, 2 out]
            n196 = Index Array(array=w322, index=0) -> (element=w319:dbl)
            n197 = property on="FileUpToDate" class="Bool (strict)"() -> ("Value"=w313:bool)  [unwired: 2 in, 2 out]
            n198 = case shown="\"CorrTubePara_SetData\"" w320 {
              tunnel: w319 -> [_ w330 w341]
              tunnel: w318 -> [_ w328 w339]
              tunnel: w317 -> [_ w327 w338]
              frame "False", Default {
              }
              frame "CorrRingPara_SetData" {
                n199 = case "Link?" shown="False" w328 {
                  tunnel: w327 -> [w333 _]
                  tunnel: [w332 UtilityLib.valueStatus."no info available" ("valueStatus")] -> w326
                  tunnel: [w331 inf] -> w329
                  tunnel: w330 -> [w331 _]
                  frame False {
                    n200 = call "CoreLib.quality 2 status.vi"("quality"=w333) -> ("valueStatus"=w332:T7)  [unwired: 18 in]
                  }
                  frame True {
                  }
                }
                n201 = control-ref of="CorrRingPara"() -> (w325:refnum<vi>)
                n202 = property class="DigNum (strict)"(reference=w325, "Value"=w329) -> ()  [unwired: 1 in, 2 out]
                n203 = call "UtilityLib.set color of GUI object.vi"("GUI object Ref"=w325, "valueStatus"=w326) -> ()  [unwired: 17 in, 1 out]
              }
              frame "CorrTubePara_SetData" {
                n204 = case "Link?" shown="False" w339 {
                  tunnel: w338 -> [w344 _]
                  tunnel: [w343 UtilityLib.valueStatus."no info available" ("valueStatus")] -> w337
                  tunnel: [w342 inf] -> w340
                  tunnel: w341 -> [w342 _]
                  frame False {
                    n205 = call "CoreLib.quality 2 status.vi"("quality"=w344) -> ("valueStatus"=w343:T7)  [unwired: 18 in]
                  }
                  frame True {
                  }
                }
                n206 = control-ref of="CorrTubePara"() -> (w336:refnum<vi>)
                n207 = property class="DigNum (strict)"(reference=w336, "Value"=w340) -> ()  [unwired: 1 in, 2 out]
                n208 = call "UtilityLib.set color of GUI object.vi"("GUI object Ref"=w336, "valueStatus"=w337) -> ()  [unwired: 17 in, 1 out]
              }
            }
            n209 = call "FileUpToDate.vi"("FileUpToDate in"=w313, "DIMControSet out"=w315, "CtlRef"=w314) -> ("FileUpToDate out"=w316:bool)  [unwired: 16 in]
            n210 = property on="FileUpToDate" class="Bool (strict)"("Value"=w316) -> ()  [unwired: 2 in, 2 out]
          }
          event "HypEndcapBTrap", "HypEndcapBInj", "HypEndcapAInj", "HypEndcapATrap", "HypEndcapAEj", "HypCorrTubeAInj", "HypCorrTubeAEj", "HypCorrTubeBInj", "HypCorrTubeBEj", "HypRing", "HypEndcapBEj": Value Change {
            # "Find sub-panel index"
            # "opening or closing a sub-panel"
            n211 = event-data() -> ("CtlRef"=w347:refnum<vi>)  [unwired: 1 in, 4 out]
            n212 = Search 1D Array(1D array=w349, element=w347) -> (index of element=w353:i32)  [unwired: 1 in]
            n213 = Index Array(array=w354, index=w353) -> (element=w351:refnum<vi>)
            n214 = invoke class="Bool" method="Reinit To Default"(reference=w347) -> ()  [unwired: 2 in, 3 out]
            n215 = property class="VI"(reference=w351) -> ("Front Panel.Open"=w350:bool)  [unwired: 1 in, 2 out]
            n216 = case "Panel Already Open?" shown="True" w350 {
              tunnel: w347 -> [w356 _]
              tunnel: w351 -> [_ w358]
              tunnel: [w355 refnum<vi> refnum ("vi reference")] -> w348
              frame False {
                n217 = call "OpenPanel.vi"("CtlRef"=w356) -> ("vi reference"=w355:refnum<vi>)  [unwired: 2 in]
              }
              frame True {
                n218 = call "PanelClose.vi"("vi reference"=w358) -> ()
              }
            }
            n219 = Replace Array Subset(array=w354, new element=w348, index=w353) -> (w352:refnum<vi>[])
          }
          event "Close All Panels": Value Change {
            n220 = event-data() -> ()  [unwired: 1 in, 6 out]
            n221 = case "Close Open Panels?" shown="True" "Close All Panels" {
              tunnel: w361 -> [w362 w364]
              tunnel: [w362 w363] -> w359
              frame False {
              }
              frame True {
                n222 = for "Close Open Panels" {
                  tunnel: w364 -> [w366] mode=indexing
                  tunnel: w364 -> [w365]
                  tunnel: [w365] -> w363
                  n223 = call "PanelClose.vi"("vi reference"=w366) -> ()
                }
              }
            }
          }
          event Timeout {
            # "Timeout"
            n224 = event-data() -> ()  [unwired: 1 in, 3 out]
          }
          event Panel Close? {
            n225 = event-data() -> ()  [unwired: 1 in, 4 out]
            n226 = stacked-sequence {
              tunnel: w372 -> [w378 _ _]
              tunnel: w371 -> [w377 _ _]
              tunnel: w370 -> [w376 _ _]
              tunnel: w369 -> [w380 _ _]
              frame #0 {
                # "Release DIM Services"
                n227 = for "Close Open Panels" {
                  tunnel: w380 -> [w390] mode=indexing
                  n228 = call "PanelClose.vi"("vi reference"=w390) -> ()
                }
                n229 = for "For Each Service" {
                  tunnel: w378 -> [w388] mode=indexing
                  n230 = Not A Number/Path/Refnum?(number/path/refnum=w388) -> (NaN/Path/Refnum?=w387:bool)
                  n231 = case "Not a Reference?" shown="False" w387 {
                    tunnel: w388 -> [w389 _]
                    frame False {
                      n232 = call "DimIndicators.dic_release_service.vi"("controlRef"=w389) -> ()  [unwired: 18 in, 1 out]
                    }
                    frame True {
                    }
                  }
                }
                n233 = for "For Each Service" {
                  tunnel: w377 -> [w385] mode=indexing
                  n234 = Not A Number/Path/Refnum?(number/path/refnum=w385) -> (NaN/Path/Refnum?=w384:bool)
                  n235 = case "Not a Reference?" shown="False" w384 {
                    tunnel: w385 -> [w386 _]
                    frame False {
                      n236 = call "DimIndicators.dic_release_service.vi"("controlRef"=w386) -> ()  [unwired: 18 in, 1 out]
                    }
                    frame True {
                    }
                  }
                }
                n237 = for "For Each Service" {
                  tunnel: w376 -> [w382] mode=indexing
                  n238 = Not A Number/Path/Refnum?(number/path/refnum=w382) -> (NaN/Path/Refnum?=w381:bool)
                  n239 = case "Not a Reference?" shown="False" w381 {
                    tunnel: w382 -> [w383 _]
                    frame False {
                      n240 = call "DimIndicators.dic_release_service.vi"("controlRef"=w383) -> ()  [unwired: 18 in, 1 out]
                    }
                    frame True {
                    }
                  }
                }
                n241 = control-ref of="Last Loaded File_Data"() -> (w379:refnum<vi>)
                n242 = control-ref of="ListOfBases_Data"() -> (w374:refnum<vi>)
                n243 = control-ref of="SetFileLocation_Data"() -> (w375:refnum<vi>)
                n244 = call "DimIndicators.dic_release_service.vi"("controlRef"=w379) -> ()  [unwired: 18 in, 1 out]
                n245 = call "DimIndicators.dic_release_service.vi"("controlRef"=w374) -> ()  [unwired: 18 in, 1 out]
                n246 = call "DimIndicators.dic_release_service.vi"("controlRef"=w375) -> ()  [unwired: 18 in, 1 out]
              }
              frame #1 {
                # "Close Front Panel"
                n247 = Current VI's Path() -> (path=w391:path)
                n248 = Open VI Reference(vi path=w391) -> (vi reference=w393:refnum<vi>, error out=w394:errorcluster)  [unwired: 5 in]
                n249 = property class="VI"(reference=w393, error in=w394, "Front Panel Window:Open"=FALSE) -> ()  [unwired: 2 out]
              }
              frame #2 {
                # "Stop Panel"
                n250 = Stop(stop? (T)=TRUE) -> ()
              }
            }
            n251 = event-data("Discard?"=TRUE) -> ()  [unwired: 1 in, 1 out]
          }
        }
      }
    }
    frame #3 {
      n252 = stacked-sequence {
        tunnel: w399 -> [w406 _ _]
        tunnel: w398 -> [w403 _ _]
        tunnel: w397 -> [w404 _ _]
        tunnel: w396 -> [w402 _ _]
        frame #0 {
          # "Release DIM Services"
          n253 = control-ref of="ListOfBases_Data"() -> (w400:refnum<vi>)
          n254 = control-ref of="SetFileLocation_Data"() -> (w401:refnum<vi>)
          n255 = control-ref of="Last Loaded File_Data"() -> (w405:refnum<vi>)
          n256 = call "DimIndicators.dic_release_service.vi"("controlRef"=w401) -> ()  [unwired: 18 in, 1 out]
          n257 = call "DimIndicators.dic_release_service.vi"("controlRef"=w405) -> ()  [unwired: 18 in, 1 out]
          n258 = call "DimIndicators.dic_release_service.vi"("controlRef"=w400) -> ()  [unwired: 18 in, 1 out]
          n259 = for "For Each Service" {
            tunnel: w404 -> [w414] mode=indexing
            n260 = Not A Number/Path/Refnum?(number/path/refnum=w414) -> (NaN/Path/Refnum?=w413:bool)
            n261 = case "Not a Reference?" shown="False" w413 {
              tunnel: w414 -> [w415 _]
              frame False {
                n262 = call "DimIndicators.dic_release_service.vi"("controlRef"=w415) -> ()  [unwired: 18 in, 1 out]
              }
              frame True {
              }
            }
          }
          n263 = for "For Each Service" {
            tunnel: w403 -> [w411] mode=indexing
            n264 = Not A Number/Path/Refnum?(number/path/refnum=w411) -> (NaN/Path/Refnum?=w410:bool)
            n265 = case "Not a Reference?" shown="False" w410 {
              tunnel: w411 -> [w412 _]
              frame False {
                n266 = call "DimIndicators.dic_release_service.vi"("controlRef"=w412) -> ()  [unwired: 18 in, 1 out]
              }
              frame True {
              }
            }
          }
          n267 = for "For Each Service" {
            tunnel: w402 -> [w408] mode=indexing
            n268 = Not A Number/Path/Refnum?(number/path/refnum=w408) -> (NaN/Path/Refnum?=w407:bool)
            n269 = case "Not a Reference?" shown="False" w407 {
              tunnel: w408 -> [w409 _]
              frame False {
                n270 = call "DimIndicators.dic_release_service.vi"("controlRef"=w409) -> ()  [unwired: 18 in, 1 out]
              }
              frame True {
              }
            }
          }
          n271 = for "Close Open Panels" {
            tunnel: w406 -> [w416] mode=indexing
            n272 = call "PanelClose.vi"("vi reference"=w416) -> ()
          }
        }
        frame #1 {
          # "Close Front Panel"
          n273 = Current VI's Path() -> (path=w420:path)
          n274 = Open VI Reference(vi path=w420) -> (vi reference=w418:refnum<vi>, error out=w417:errorcluster)  [unwired: 5 in]
          n275 = property class="VI"(reference=w418, error in=w417, "Front Panel Window:Open"=FALSE) -> ()  [unwired: 2 out]
        }
        frame #2 {
          # "Stop Panel"
          n276 = Stop(stop? (T)=TRUE) -> ()
        }
      }
    }
  }
  n277 = call "LVDimInterface.dim_operate.vi"("DNSNode"="lebit-balcony") -> ()  [unwired: 19 in]
